vi "3.4.vi"(2 "字符串 2":string, 3 "输入 1":dbl, 4 "字符串":string) -> (0 "长度":i32, 1 "连接的字符串":string)   [LabVIEW 2017]
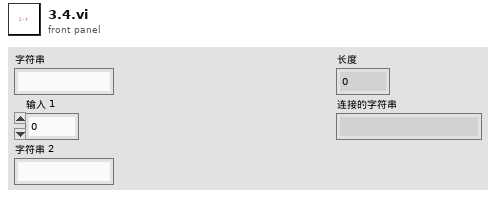
[diagram p1: front panel]
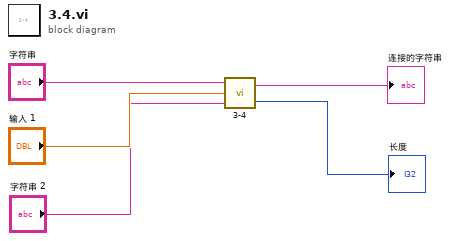
[diagram p0: block diagram]
diagram:
  n1 = call "3-4.vi"("字符串 2"="字符串 2", "输入 1"="输入 1", "字符串"="字符串") -> ("长度"=→"长度":i32, "连接的字符串"=→"连接的字符串":string)
